vi "Init Device.vi"(8 "error in (no error)":errorcluster, 11 "TE2000 in":refnum<class "TE2000.lvclass">) -> (0 "error out":errorcluster, 3 "TE2000 out":refnum<class "TE2000.lvclass">)   [LabVIEW 2014, in "TE2000.lvlib" / "TE2000.lvclass"]
uses:
  TE2000.lvclass
  TE2000.lvclass/TE2000.ctl
  <vilib>/Instr/_visa.llb/VISA Configure Serial Port (Instr).vi
  Device/Device.lvclass
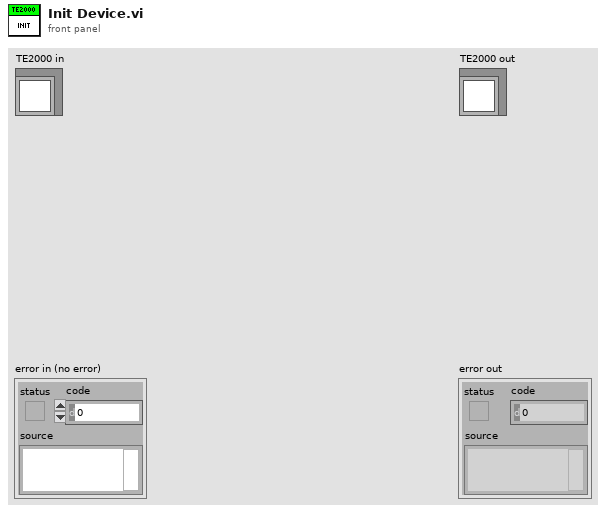
[diagram p1: front panel]
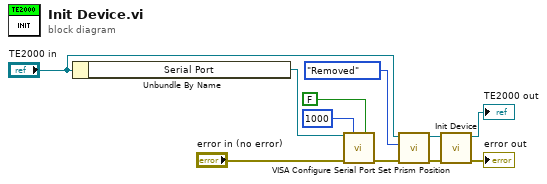
[diagram p0: block diagram]
diagram:
  n1 = Unbundle By Name("TE2000 in") -> ("Serial Port"=w7:refnum<visa-resource-name>)
  n2 = call-poly "VISA Configure Serial Port"("VISA resource name"=w7, "timeout (10sec)"=u32 1000, "Enable Termination\nChar (T)"=FALSE ("Enable Termination\nChar (T)"), "error in (no error)"="error in (no error)") -> ("error out"=w4:errorcluster)  [unwired: 10 in, 1 out]
  n3 = call-dynamic "Set Prism Position.vi"("error in (no error)"=w4, "Prism Position"=enum16{"Removed", "Inserted"}."Removed", "TE2000 in"="TE2000 in") -> ("error out"=w1:errorcluster, "TE2000 out"=w2:refnum<class "TE2000.lvclass">)  [unwired: 7 in]
  n4 = call-parent "Init Device.vi"("error in (no error)"=w1, "Device in"=w2) -> ("error out"=→"error out":errorcluster, "Device out"=→"TE2000 out":refnum<class "TE2000.lvclass">)  [unwired: 8 in]
